vi "process_error.vi"(8 "error in (no error)":errorcluster, 9 "Update Status":bool, 10 "No Error Message":string, 11 "lightfield_panel in":refnum<class "lightfield_panel.lvclass">) -> (0 "error out":errorcluster, 3 "lightfield_panel out":refnum<class "lightfield_panel.lvclass">)   [LabVIEW 2015, in "lightfield_panel.lvclass"]
uses:
  lightfield_panel.lvclass
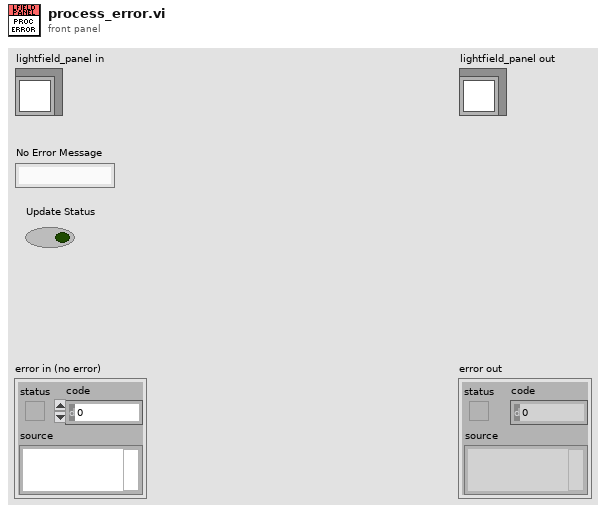
[diagram p1: front panel]
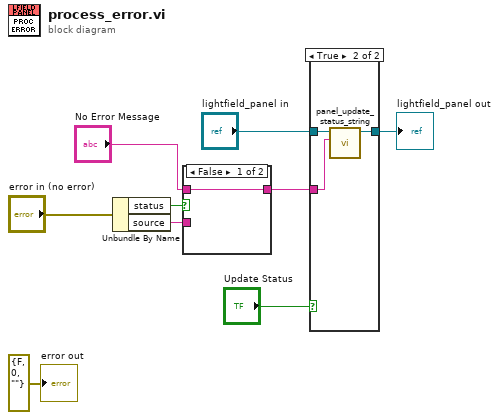
[diagram p0: block diagram]
diagram:
  n1 = Unbundle By Name("error in (no error)") -> ("status"=w9:bool, "source"=w7:string)
  n2 = case shown="False" w9 {
    tunnel: "No Error Message" -> [w10 _]
    tunnel: [w10 w11] -> w8
    tunnel: w7 -> [_ w11]
    frame False {
    }
    frame True {
    }
  }
  n3 = case shown="True" "Update Status" {
    tunnel: "lightfield_panel in" -> [w12 w15]
    tunnel: w8 -> [_ w14]
    tunnel: [w12 w13] -> w1
    frame False {
    }
    frame True {
      n4 = call-dynamic "panel_update_status_string.vi"("String"=w14, "lightfield_panel in"=w15) -> ("lightfield_panel out"=w13:refnum<class "lightfield_panel.lvclass">)  [unwired: 8 in, 1 out]
    }
  }
  "lightfield_panel out" <- w1
  "error out" <- errorcluster {"status"=FALSE, "code"=0, "source"=""} ("error out")
